vi "Test TDMS store recall.vi"() -> ()   [LabVIEW 2016]
uses:
  <vilib>/Utility/Data Type/Type Definitions/Data Type.ctl
  <vilib>/Utility/Data Type/Type Definitions/Type Definition Info.ctl
  <vilib>/Utility/Data Type/NI_Data Type.lvlib
panel:
  out "Value out":variant
  out "Parameter out":timestamp
  in  "File Path Control":path=path "C:/Data/test.tdms"
  out "Type Definition Info":T1
  out "Type Definition":bool
  out "Name":string
  out "Type":T2
  in  "Parameter":cluster{"Numeric Control":dbl, "Boolean":bool}
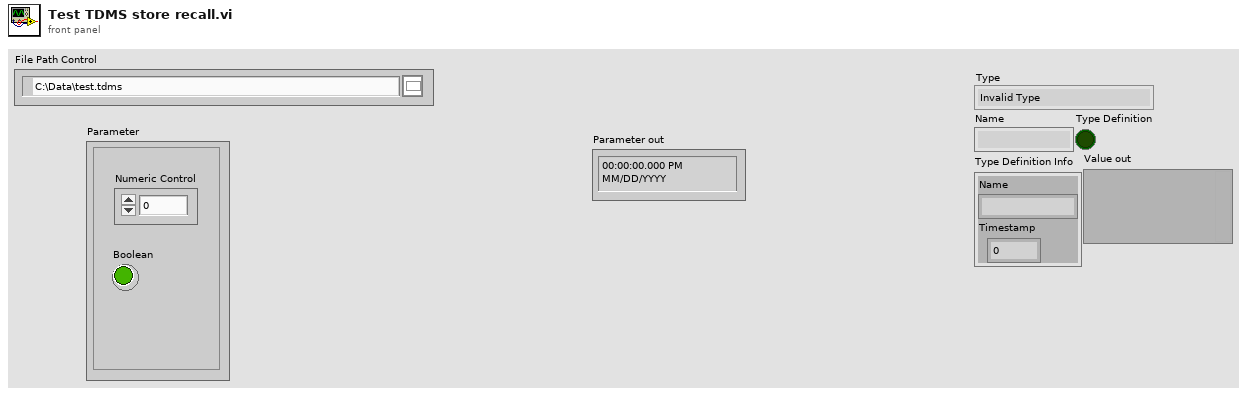
[diagram p1: front panel]
types:
  T1 = typedef "NI_Data Type.lvlib/Type Definition Info.ctl" = cluster{"Name":string, "Timestamp":u32}
  T2 = typedef "NI_Data Type.lvlib/Data Type.ctl" = enum8{"Invalid Type", "Void", "I8", "I16", "I32", "I64", "U8", "U16", "U32", "U64", "Single Float", "Double Float", "Extended Float", "Single Complex", "Double Complex", "Extended Complex", "Enum U8", "Enum U16", "Enum U32", "Enum U64", "Single Float With Unit", "Double Float With Unit", "Extended Float With Unit", "Single Complex with Unit", "Double Complex with Unit", "Extended Complex with Unit", "Boolean", "String", "Path", "Picture", "Tag", "Array", "Cluster", "Variant", "LV Variant", "Waveform", "Timestamp", "Digital Waveform", "Digital Data", "ExpressData", "Refnum", "External Data", "VI", "Poly VI", "LabVIEW Class Instance", "Fixed Point"}
  T3 = enum16{"open", "open or create", "create or replace", "create", "open (read-only)"}
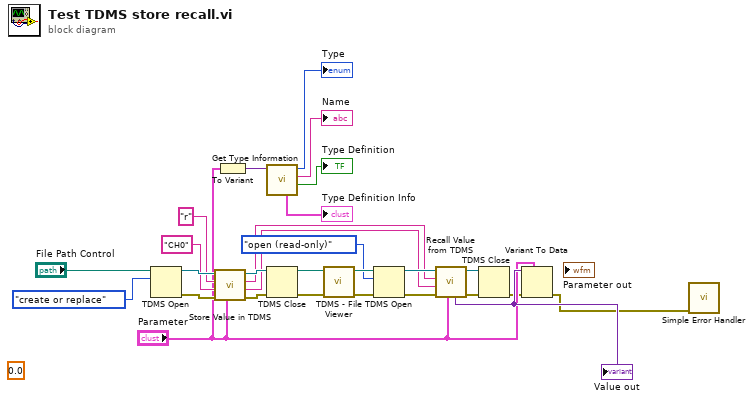
[diagram p0: block diagram]
diagram:
  (unwired) 0.0 ("Numeric Control")
  n1 = TDMS Open(10:T3."create or replace" ("operation (0:open)"), 11:"File Path Control") -> (0:w20:errorcluster, 3:w22:refnum<k34>)  [unwired: 5 in]
  n2 = call "Store Value in TDMS.vi"("Value"="Parameter", "Error In"=w20, "channel name"="CH0", "group name"="r", "tdms file"=w22) -> ("Error Out"=w17:errorcluster, "channel name out"=w2:string, "group name out"=w3:string, "tdms file out"=w16:refnum<k34>)  [unwired: 3 in]
  n3 = To Variant(anything="Parameter") -> (Variant=w28:variant)
  n4 = call <vilib>:"Get Type Information.vi"("Variant"=w28) -> ("Type Definition"=→"Type Definition":bool, "Name"=→"Name":string, "Type"=→"Type":T2, "Type Definition Info"=→"Type Definition Info":T1)  [unwired: 6 in, 1 out]
  n5 = TDMS Close(8:w17, 11:w16) -> (0:w15:errorcluster, 3:w14:path)
  n6 = call <vilib>:"TDMS - File Viewer.vi"("error in (no error)"=w15, "file path"=w14) -> ("error out"=w12:errorcluster, "file path out"=w11:path)  [unwired: 4 in]
  n7 = TDMS Open(8:w12, 10:T3."open (read-only)" ("operation (0:open)"), 11:w11) -> (0:w4:errorcluster, 3:w8:refnum<k34>)  [unwired: 4 in]
  n8 = call "Recall Value from TDMS.vi"("Value"="Parameter", "Error In"=w4, "channel name"=w2, "group name"=w3, "tdms file"=w8) -> ("Error Out"=w7:errorcluster, "tdms file out"=w5:refnum<k34>, "Value out"=w13:variant)  [unwired: 2 in, 2 out]
  "Value out" <- w13
  n9 = TDMS Close(8:w7, 11:w5) -> (0:w6:errorcluster)  [unwired: 1 out]
  n10 = Variant To Data(error in=w6, type="Parameter", Variant=w13) -> (error out=w1:errorcluster)  [unwired: 1 out]
  n11 = call <vilib>:"Simple Error Handler.vi"("error in (no error)"=w1) -> ()  [unwired: 4 in, 5 out]
